vi "TestMatlabConvertTimeThroughTempValue.vi"() -> ()   [LabVIEW 2017]
panel:
  out "Convert to matlab param":timestamp
  out "Totals info":i32(listbox)
  out "Single read info":i32(listbox)
  out "Read data":variant
  out "Data":variant
  out "Temp Index":dbl
  out "erros?":bool
  out "ExpID":string="Exp77c27ca2690b43b31b68791e85e1b449C"
  out "Read temp values":timestamp
  out "Read size":i32
  out "Set temp values":timestamp
  out "Start":timestamp
  in  "MatrixSIze":dbl=1000.0
  in  "# Iterations":i32=100
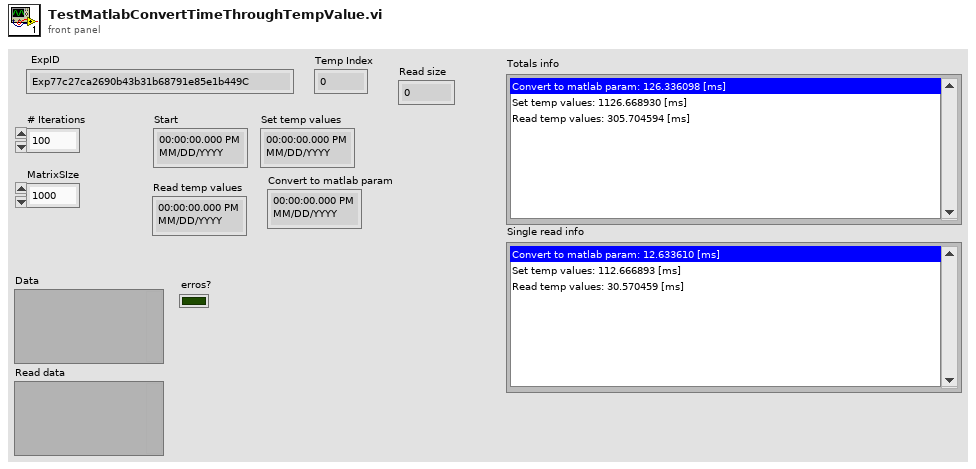
[diagram p1: front panel]
types:
  T1 = typedef "MatlabDataBundle.ctl" = cluster{"MatlabType":T2, "Value":variant, "Name":string, "Typename":string, "Container Type":T3}
  T2 = typedef "MatlabDataType.ctl" = enum16{"NotAMatlabType", "Real", "Complex", "String", "Boolean"}
  T3 = typedef "MatlabDataContainerType.ctl" = enum16{"Numeric Value", "Numeric Array", "Waveform"}
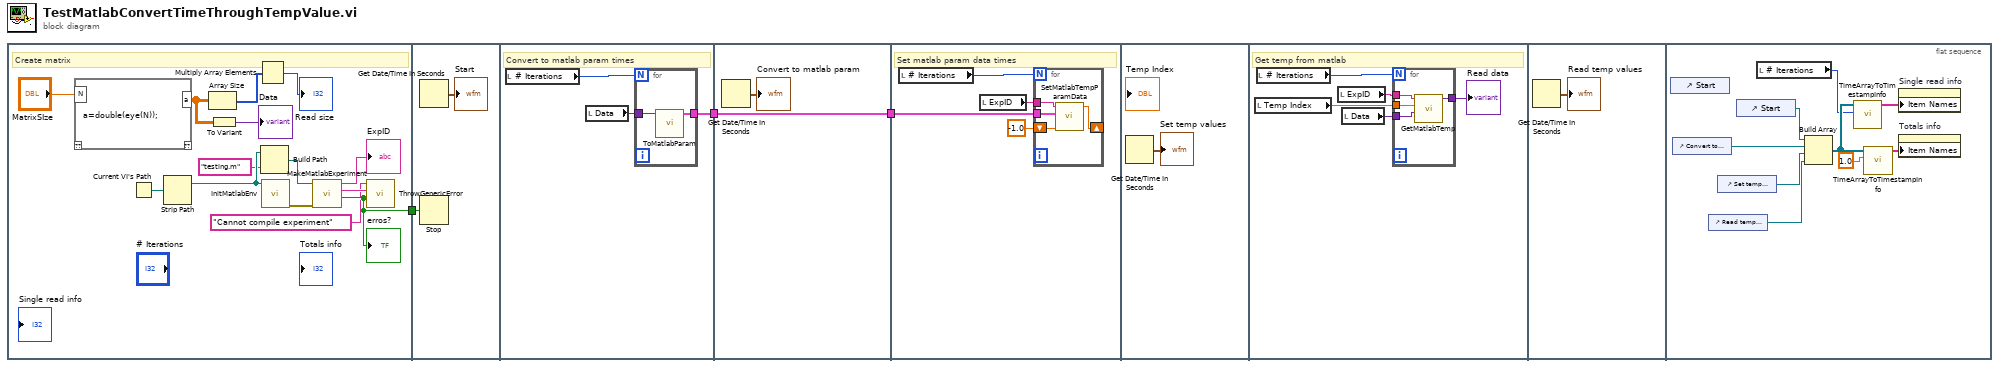
[diagram p0: block diagram]
diagram:
  n1 = flat-sequence {
    tunnel: [w6] -> w3
    tunnel: w3 -> [w18]
    tunnel: [w20] -> w2
    tunnel: w2 -> [w26]
    tunnel: [w26] -> w1
    tunnel: w1 -> [w30]
    frame #0 {
      # "Create matrix"
      n2 = script code="a=double(eye(N));"("N"="MatrixSIze") -> ("a"=w9:dbl[][])  [unwired: 1 in, 1 out]
      n3 = Current VI's Path() -> (path=w13:path)
      n4 = Strip Path(path=w13) -> (stripped path=w15:path)  [unwired: 1 out]
      n5 = Array Size(array=w9) -> (size(s)=w8:i32[])
      n6 = To Variant(anything=w9) -> (Variant=→"Data":variant)
      n7 = Multiply Array Elements(1:w8) -> (0:→"Read size":i32)
      n8 = Build Path(base path=w15, name or relative path="testing.m") -> (appended path=w16:path)
      n9 = call "InitMatlabEnv.vi"("Working directory"=w15) -> ("error out"=w14:errorcluster)  [unwired: 10 in]
      n10 = call "MakeMatlabExperiment.vi"("error in"=w14, "experimentFilepath"=w16) -> ("erros?"=w6:bool, "errors"=w5:string, "ExpID"=→"ExpID":string)  [unwired: 6 in, 1 out]
      "erros?" <- w6
      n11 = call "ThrowGenericError.vi"("Invoke?"=w6, "Error info"=w5, "TheError"="Cannot compile experiment") -> ()  [unwired: 8 in, 1 out]
    }
    frame #1 {
      n12 = Get Date/Time In Seconds() -> (seconds since 1Jan1904=→"Start":timestamp)
      n13 = Stop(stop? (T)=w18) -> ()
    }
    frame #2 {
      # "Convert to matlab param times"
      n14 = local read "# Iterations"() -> (w22:i32)
      n15 = local read "Data"() -> (w21:variant)
      n16 = for {
        N: w22 -> [_]
        tunnel: w21 -> [w24]
        tunnel: [w23] -> w20
        n17 = call "ToMatlabParam.vi"("Value"=w24) -> ("Matlab Param Data"=w23:T1[])  [unwired: 10 in]
      }
    }
    frame #3 {
      n18 = Get Date/Time In Seconds() -> (seconds since 1Jan1904=→"Convert to matlab param":timestamp)
    }
    frame #4 {
      # "Set matlab param data times"
      n19 = local read "# Iterations"() -> (w27:i32)
      n20 = local read "ExpID"() -> (w28:string)
      n21 = for {
        N: w27 -> [_]
        tunnel: w30 -> [w34]
        shift-right: [w32] -> _
        shift-left: -1.0 ("Temp Index") -> [w33]
        tunnel: w28 -> [w31]
        n22 = call "SetMatlabTempParamData.vi"("index in"=w33, "Matlab param data"=w34, "ExperimentID"=w31) -> ("index out"=w32:dbl)  [unwired: 8 in]
      }
    }
    frame #5 {
      n23 = Get Date/Time In Seconds() -> (seconds since 1Jan1904=→"Set temp values":timestamp)
    }
    frame #6 {
      # "Get temp from matlab"
      n24 = local read "Temp Index"() -> (w38:dbl)
      n25 = local read "# Iterations"() -> (w40:i32)
      n26 = local read "ExpID"() -> (w39:string)
      n27 = local read "Data"() -> (w37:variant)
      n28 = for {
        N: w40 -> [_]
        tunnel: w39 -> [w44]
        tunnel: w38 -> [w43]
        tunnel: w37 -> [w42]
        tunnel: [w41] -> w36
        n29 = call "GetMatlabTemp.vi"("Value To Update (or type)"=w42, "index in"=w43, "ExpID"=w44) -> ("Value"=w41:variant)  [unwired: 6 in, 2 out]
      }
      "Read data" <- w36
    }
    frame #7 {
      n30 = Get Date/Time In Seconds() -> (seconds since 1Jan1904=→"Read temp values":timestamp)
    }
    frame #8 {
      n31 = control-ref of="Start"() -> ()  [unwired: 1 out]
      n32 = control-ref of="Convert to matlab param"() -> (w51:refnum<vi>)
      n33 = control-ref of="Read temp values"() -> (w49:refnum<vi>)
      n34 = control-ref of="Set temp values"() -> (w50:refnum<vi>)
      n35 = control-ref of="Start"() -> (w52:refnum<vi>)
      n36 = local read "# Iterations"() -> (w47:i32)
      n37 = Build Array(w52, w51, w50, w49) -> (w48:refnum<vi>[])
      n38 = call "TimeArrayToTimestampInfo.vi"("Number of iterations"=w47, "Times array in"=w48) -> ("Array out"=w53:string[])  [unwired: 9 in]
      n39 = call "TimeArrayToTimestampInfo.vi"("Number of iterations"=1.0, "Times array in"=w48) -> ("Array out"=w54:string[])  [unwired: 9 in]
      n40 = property on="Single read info" class="LstBox (strict)"("Item Names"=w53) -> ()  [unwired: 2 in, 2 out]
      n41 = property on="Totals info" class="LstBox (strict)"("Item Names"=w54) -> ()  [unwired: 2 in, 2 out]
    }
  }
